vi "Read Permissions.vi"(8 "Error In":errorcluster, 11 "File Info In":refnum<class "File Info.lvclass">) -> (0 "Error Out":errorcluster, 2 "Permissions":T1, 3 "File Info Out":refnum<class "File Info.lvclass">)   [LabVIEW 2018, in "Toolkit.lvlib" / "File Info.lvclass"]
uses:
  File Info.lvclass
  Typedefs/Permissions.ctl
  Typedefs/Modes.ctl
  File Info.lvclass/File Info.ctl
  SSH/SSH.lvclass/SSH.ctl
  Toolkit.lvlib
  SSH/SSH.lvclass
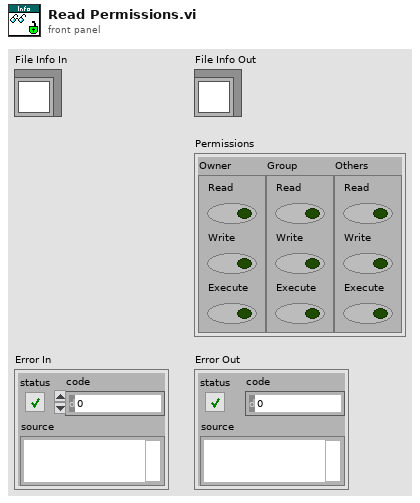
[diagram p1: front panel]
types:
  T1 = typedef "Toolkit.lvlib/Permissions.ctl" = cluster{"Owner":T2, "Group":T2, "Others":T2}
  T2 = typedef "Toolkit.lvlib/Modes.ctl" = cluster{"Read":bool, "Write":bool, "Execute":bool}
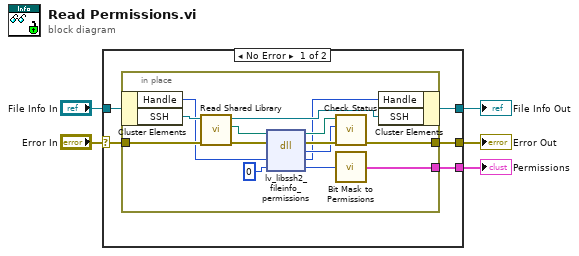
[diagram p0: block diagram]
diagram:
  n1 = case shown="No Error" "Error In" {
    selector: "Error In" -> [w9 w26]
    tunnel: [w7 w26] -> w4
    tunnel: "File Info In" -> [w10 w25]
    tunnel: [w8 w25] -> w2
    tunnel: [w6 _] -> w1
    frame No Error {
      n2 = in-place {
        in-place-border: w9 -> [w17]
        in-place-border: [w14] -> w7
        in-place-border: [w11] -> w6
        n3 = in-place-cluster #1(w10) -> ("Handle"=w16:u64, "SSH"=w21:refnum<class "SSH.lvclass">)
        n4 = call "Read Shared Library.vi"("Error In"=w17, "SSH In"=w21) -> ("Error Out"=w18:errorcluster, "lv-libssh2 Shared Library"=w19:path, "SSH Out"=w20:refnum<class "SSH.lvclass">)  [unwired: 7 in]
        n5 = dll-call lib="lv-libssh2.*" fn="lv_libssh2_fileinfo_permissions"(path in=w19, error in=w18, "handle"=w16, "permissions"=u32 0 ("flags")) -> (path out=w23:path, error out=w24:errorcluster, "status"=w22:i32, "handle"=w15:u64, "permissions"=w12:u32)  [unwired: 1 in]
        n6 = call "Check Status.vi"("Error In"=w24, "Status"=w22, "lv-libssh2 Shared Library In"=w23) -> ("Error Out"=w14:errorcluster)  [unwired: 7 in, 1 out]
        n7 = call "Bit Mask to Permissions.vi"("Bit Mask"=w12) -> ("Permissions"=w11:T1)
        n8 = in-place-cluster #1("Handle"=w15, "SSH"=w20) -> (w8:refnum<class "File Info.lvclass">)
      }
    }
    frame Error {
    }
  }
  "Error Out" <- w4
  "File Info Out" <- w2
  "Permissions" <- w1
